vi "licdf get info.vi"(0 "handle":i32, 1 "out_proto_major":i32, 2 "out_proto_minor":i32, 3 "out_fw_major":i32, 4 "out_fw_minor":i32, 5 "out_fw_patch":i32, 6 "out_flags":i32, 7 "error in (no error)":errorcluster, 8 "out_capacity":i32, 9 "out_free":i32) -> (18 "out_capacity out":i32, 19 "out_free out":i32, 20 "function return":i32, 21 "out_proto_major out":i32, 22 "out_proto_minor out":i32, 23 "out_fw_major out":i32, 24 "out_fw_minor out":i32, 25 "out_fw_patch out":i32, 26 "out_flags out":i32, 27 "error out":errorcluster)   [LabVIEW 2026, in "keynub_licdongle.lvlib"]
doc: "int32_t licdf_get_info(int32_t handle, int32_t *out_proto_major, int32_t *out_proto_minor,\n int32_t *out_fw_major, int32_t *out_fw_minor, int32_t *out_fw_patch,\n int32_t *out_flags, int32_t *out_capacity, int32_t *out_free);"
uses:
  keynub_licdongle.lvlib
  natives/win-x64/keynub_licdongle_flat.dll
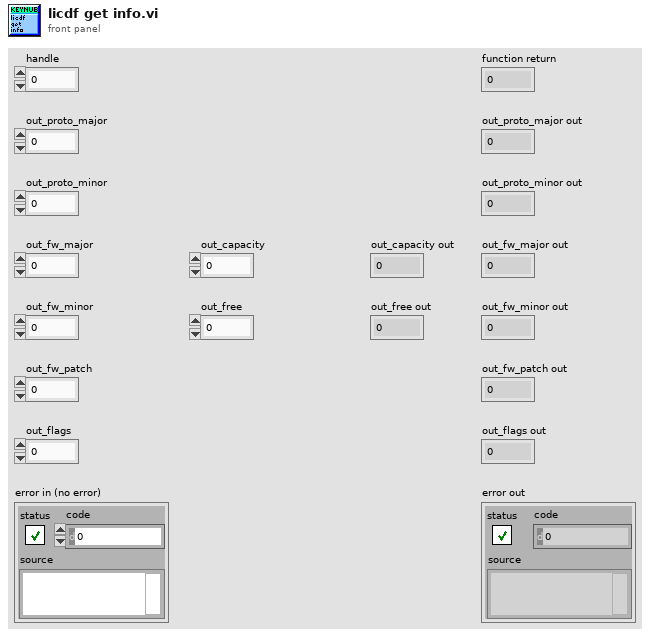
[diagram p1: front panel]
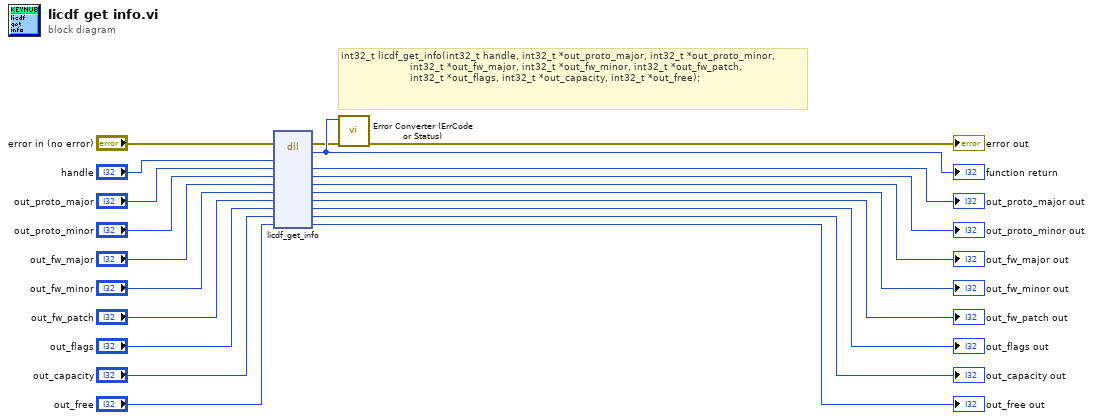
[diagram p0: block diagram]
diagram:
  # "int32_t licdf_get_info(int32_t handle, int32_t *out_proto_major, int32_t *out_proto_minor,\n                       int32_t *out_fw_major, int32_t *out_fw_minor, int32_t *out_fw_patch,\n                       int32_t *out_flags, int32_t *out_capacity, int32_t *out_free);"
  n1 = dll-call lib="C:/Austausch/KeyNub/LicenseDongle-PublicSDK/natives/win-x64/keynub_licdongle_flat.*" fn="licdf_get_info"(error in="error in (no error)", "handle"="handle", "out_proto_major"="out_proto_major", "out_proto_minor"="out_proto_minor", "out_fw_major"="out_fw_major", "out_fw_minor"="out_fw_minor", "out_fw_patch"="out_fw_patch", "out_flags"="out_flags", "out_capacity"="out_capacity", "out_free"="out_free") -> (error out=w2:errorcluster, w21:i32, "out_proto_major"=→"out_proto_major out":i32, "out_proto_minor"=→"out_proto_minor out":i32, "out_fw_major"=→"out_fw_major out":i32, "out_fw_minor"=→"out_fw_minor out":i32, "out_fw_patch"=→"out_fw_patch out":i32, "out_flags"=→"out_flags out":i32, "out_capacity"=→"out_capacity out":i32, "out_free"=→"out_free out":i32)  [unwired: 3 in, 1 out]
  "function return" <- w21
  n2 = call "Error Converter (ErrCode or Status).vi"("error in (no error)"=w2, "error code"=w21) -> ("error out"=→"error out":errorcluster)  [unwired: 9 in]
